vi "STS_spectroscopy_V1.vi"(6 "Internal use":string, 7 "Grid param":T1 {"height (m)" format="%#_6p"; "width (m)" format="%#_6p"; "center Y (m)" format="%#_6p"; "center X (m)" format="%#_6p"}, 8 "Error in (no error)":errorcluster, 9 "Points Y/Index Y":i32, 10 "Points X/Index X":i32, 11 "Method":enum16{"init", "run", "end"}(ring)=enum."end") -> (0 "Error out":errorcluster)   [LabVIEW 2014]
doc: "Example of a measurement VI to be used in the \"Experiments on a Grid\" tool as external VI.\n\nThis example measure the topography and spectroscopy data. The spectroscopy measurements are taken on a subgrid. The data are saved to a sxm and a binary file.\n\n- Nanonis Programming Interface -"
uses:
  <userlib>/Nanonis Prog Interface V5/Scan/Grid/LinePatternGet.vi
  <userlib>/Nanonis Prog Interface V5/Scan/Grid/GridPatternGet.vi
  <userlib>/Nanonis Prog Interface V5/Scan/Grid/CloudPatternGet.vi
  <userlib>/Nanonis Prog Interface V5/Nanonis Prog Interface.lvlib
panel:
  out "Status 2":string="finishing"
  in  "Lockin delay [ms]":u32
  in  "Z Controller ON/OFF":bool
  in  "type":u16(ring)=1 items=["Line", "Grid", "Cloud"]
  in  "Lockin ON/OFF":bool
  in  "Correct Drift":bool=TRUE
  in  "Email when finished":string="cornelius.krull@monash.edu, dhaneesh.gopalakrishnan@monash.edu"
  in  "STS z offset":dbl format="%#_6p"
  out "ETA":timestamp=timestamp(3582621546.85837 s since 1904-01-01)
  out "remaining":dbl=19834.093046092985 format="%<%H:%M:%S>t"
  out "Progress":u8(slide)=5 scale=0.0..100.0 scale format="%#.1g"
  out "total Points":i32=576
  in  "preSTS delay [ms]":u32=3
  in  "STS Bias":dbl=-3.4 format="%#_6p"
  in  "Move Bias":dbl=-3.4 format="%#_6p"
  in  "Move Current":dbl=5e-11 format="%#_6p"
  in  "Imaging Bias":dbl=-3.4 format="%#_6p"
  in  "max applied Drift Correction":i32=20 min=1 max=100 step=1 format="%.0p"
  in  "Correlate":u16(ring) items=["first Frame", "successive Frames"]
  out "Topo Images taken":i32
  in  "Increment":i32=40
  in  "Threshold":i32=2 min=1 step=1
  in  "tip Speed (m/s)":sgl=1e-08 format="%.2p"
  out "X drift":i32
  out "Y drift":i32
  out "Last Drift detected":i32
  in  "MaxImagesBack":i32=2
  in  "Channel index (0-23)":u8(ring) items=["Current"=0, "Z (m)"=14]
  in  "File name":string="DCA_cluster_STS_Grid"
  in  "STS Current":dbl=5e-11 format="%#_6p"
  in  "Imaging Current":dbl=5e-11 format="%#_6p"
  in  "zdrift \nDuration (s)":dbl
  in  "Correct z drift":bool
  out "Status":string="finishing"
  in  "Drift correction Pixels":i32=256 caption="Topo Pixels"
  out "Y Offset":dbl format="%#_6p"
  out "X Offset":dbl format="%#_6p"
  out "Points taken":dbl=30.0
  in  "Drift Correction every":i32=40
  in  "Y subgrid spacing":u16=1
  in  "X subgrid spacing":u16=1
  # "GRID points"
  # "Increase this if no Drift was detected for \na certain number of images"
  # "%"
  # "time (HH:MM:SS)"
  # "images back"
  # "% of image size"
  # "<--Z Cont. Needs to be off"
  # "RUN smart tilt before starting the GRID | Img Angle = 0"
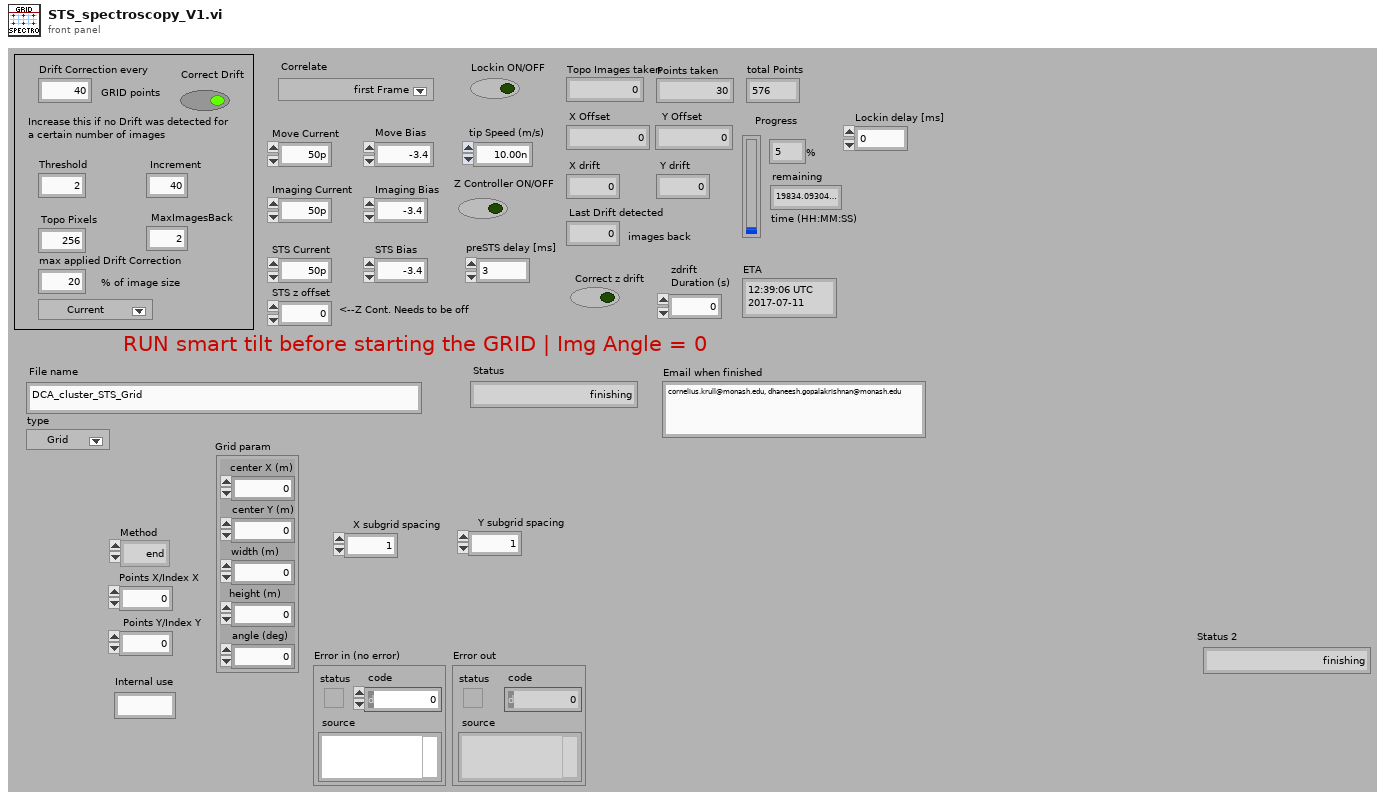
[diagram p1: front panel]
types:
  T1 = cluster{"center X (m)":sgl, "center Y (m)":sgl, "width (m)":sgl, "height (m)":sgl, "angle (deg)":sgl}
  T2 = cluster{"Drift correction Pixels":i32, "Imaging Current":dbl, "STS Current":dbl, "MaxImagesBack":i32, "tip Speed (m/s)":sgl, "Threshold":i32, "Increment":i32, "Correlate":u16, "max applied Drift Correction":i32, "Imaging Bias":dbl, "Move Current":dbl, "Move Bias":dbl, "STS Bias":dbl, "preSTS delay [ms]":u32, "STS z offset":dbl, "Correct Drift":bool, "Lockin ON/OFF":bool}
  T3 = cluster{"center X":sgl, "center Y":sgl, "angle":sgl, "width":sgl, "height":sgl, "# pixels":i32, "# lines":i32}
  T4 = cluster{"Name":string, "Calibration":sgl, "Offset":sgl, "Channel index":i32}[]
  T5 = cluster{"up/down":bool, "time/line":sgl, "start time":timestamp, "end time":timestamp}
  T6 = cluster{"Z averaging time (s)":sgl, "Z offset (m)":sgl, "Initial settling time (s)":sgl}
  T7 = cluster{"Max. slew rate (V/s)":sgl, "Settling time (s)":sgl, "Integration time (s)":sgl}
  T8 = cluster{"End settling time (s)":sgl, "Z control time (s)":sgl}
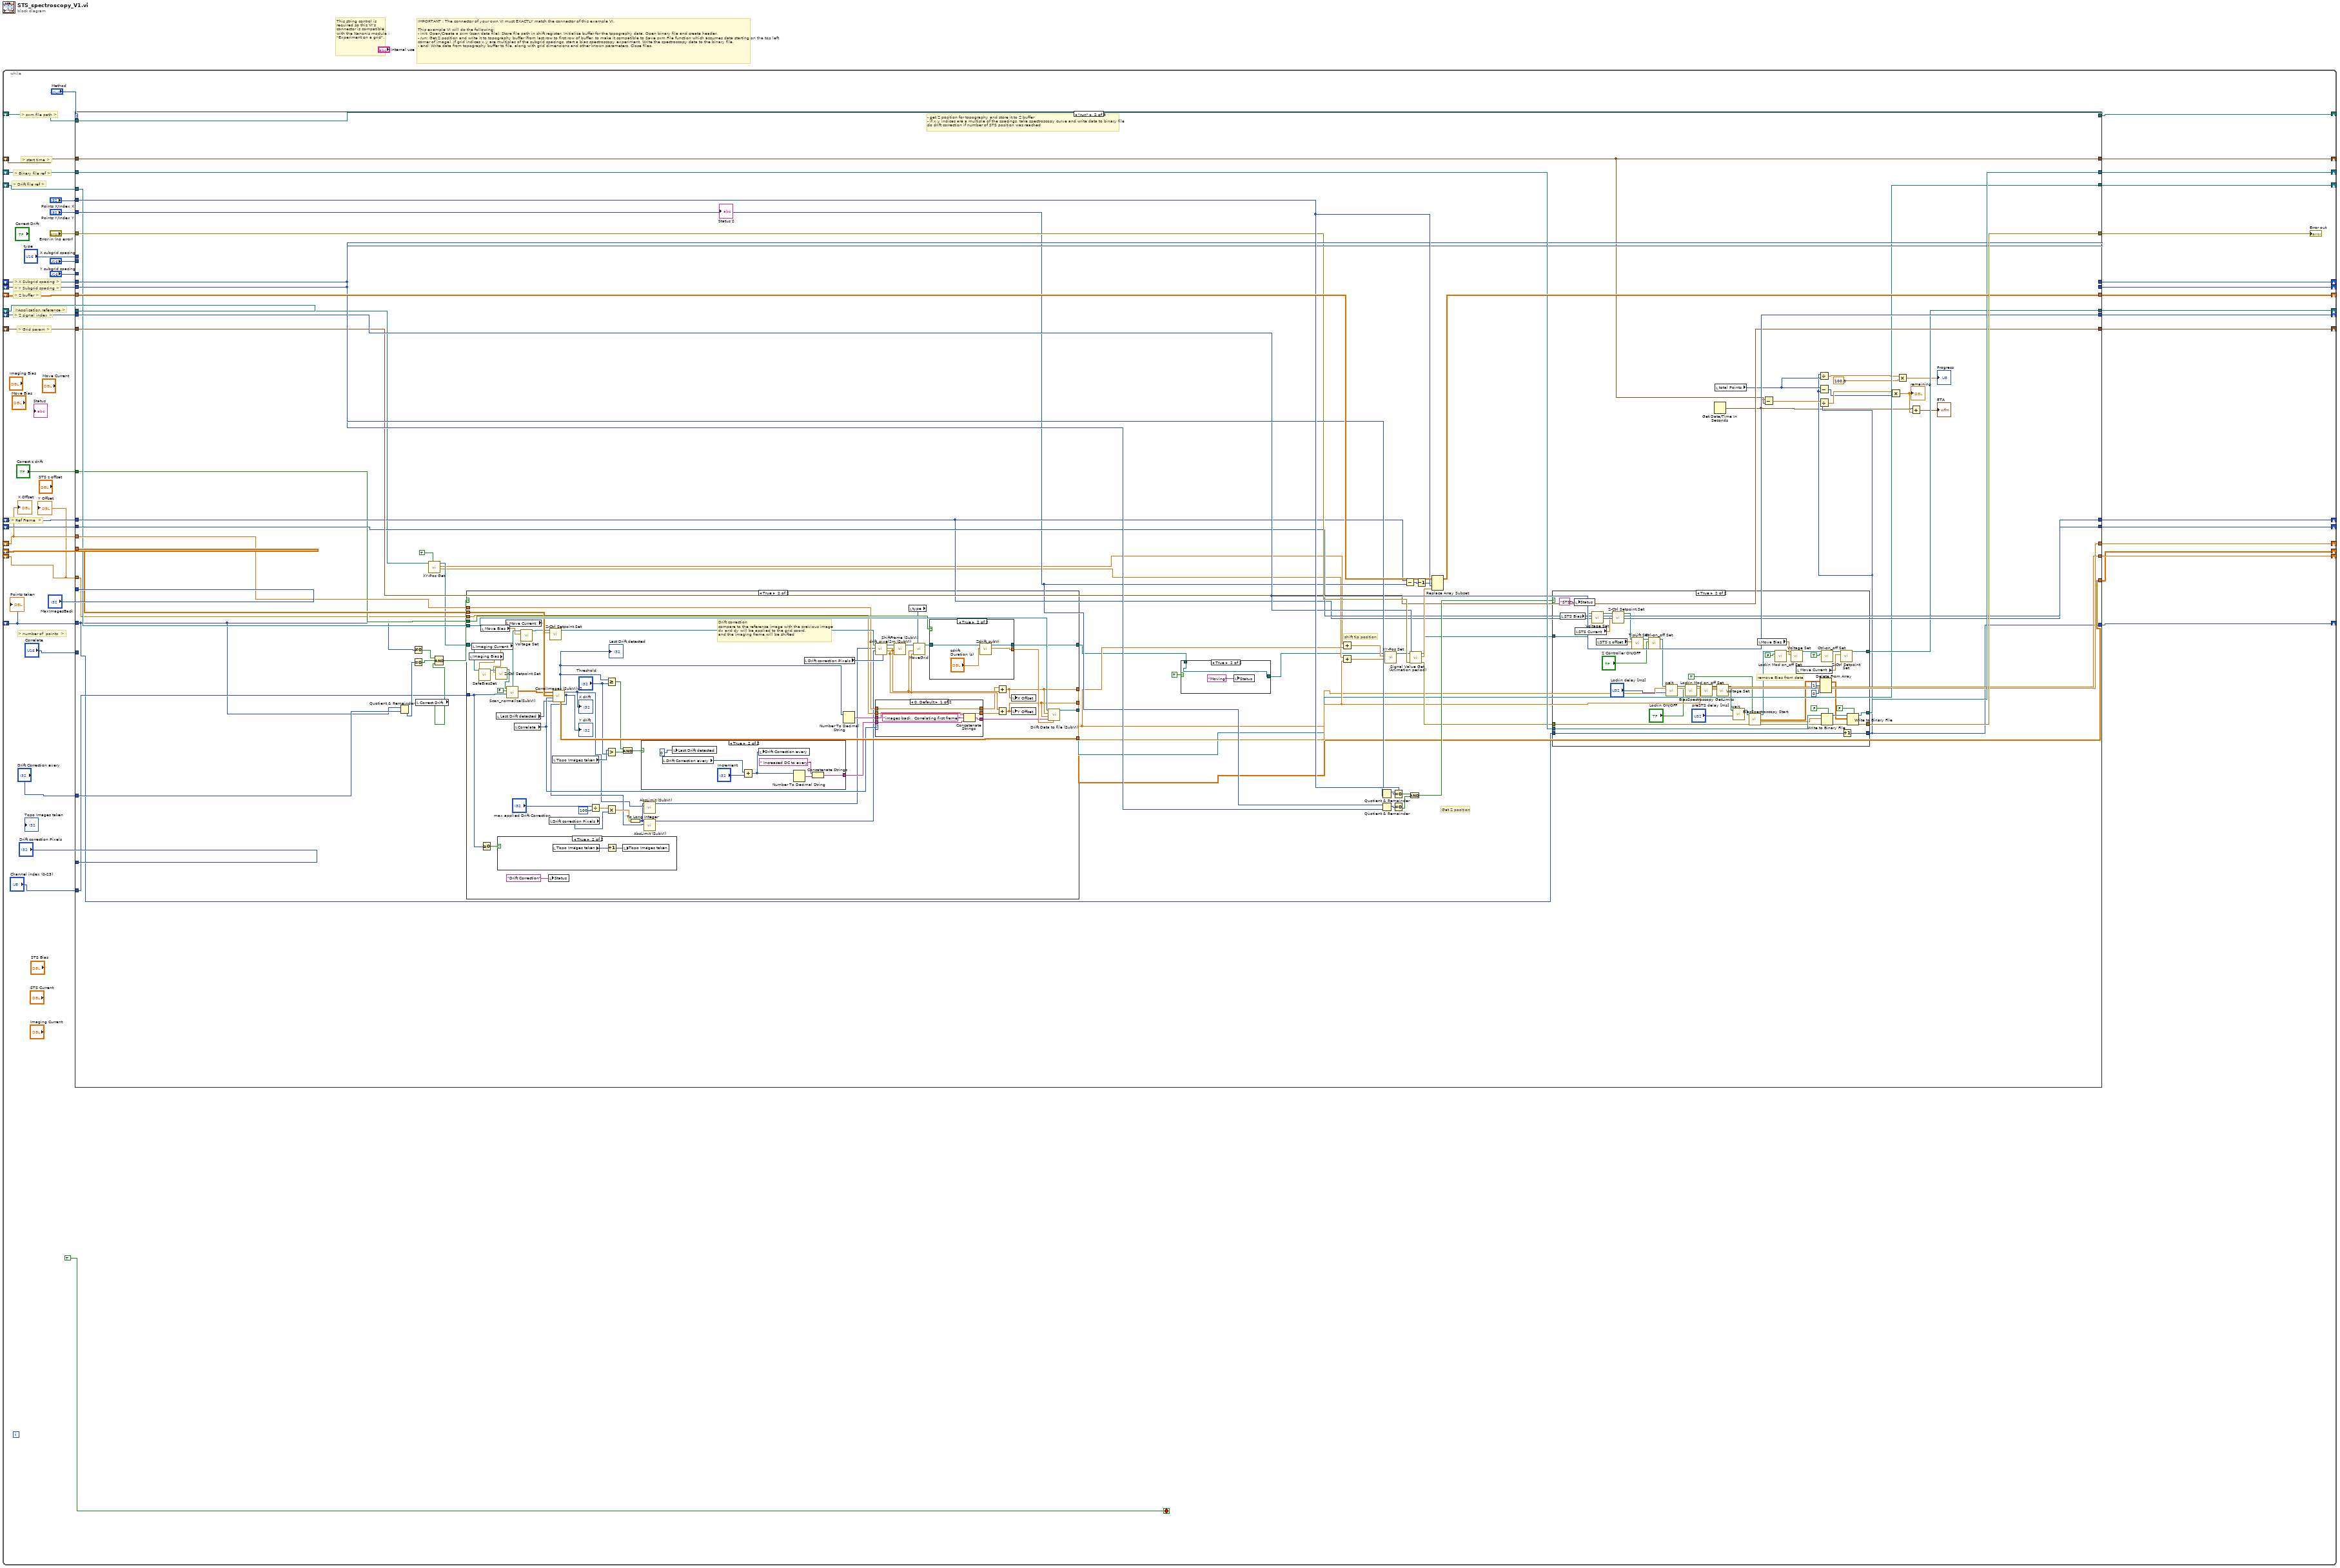
[diagram p0: block diagram]
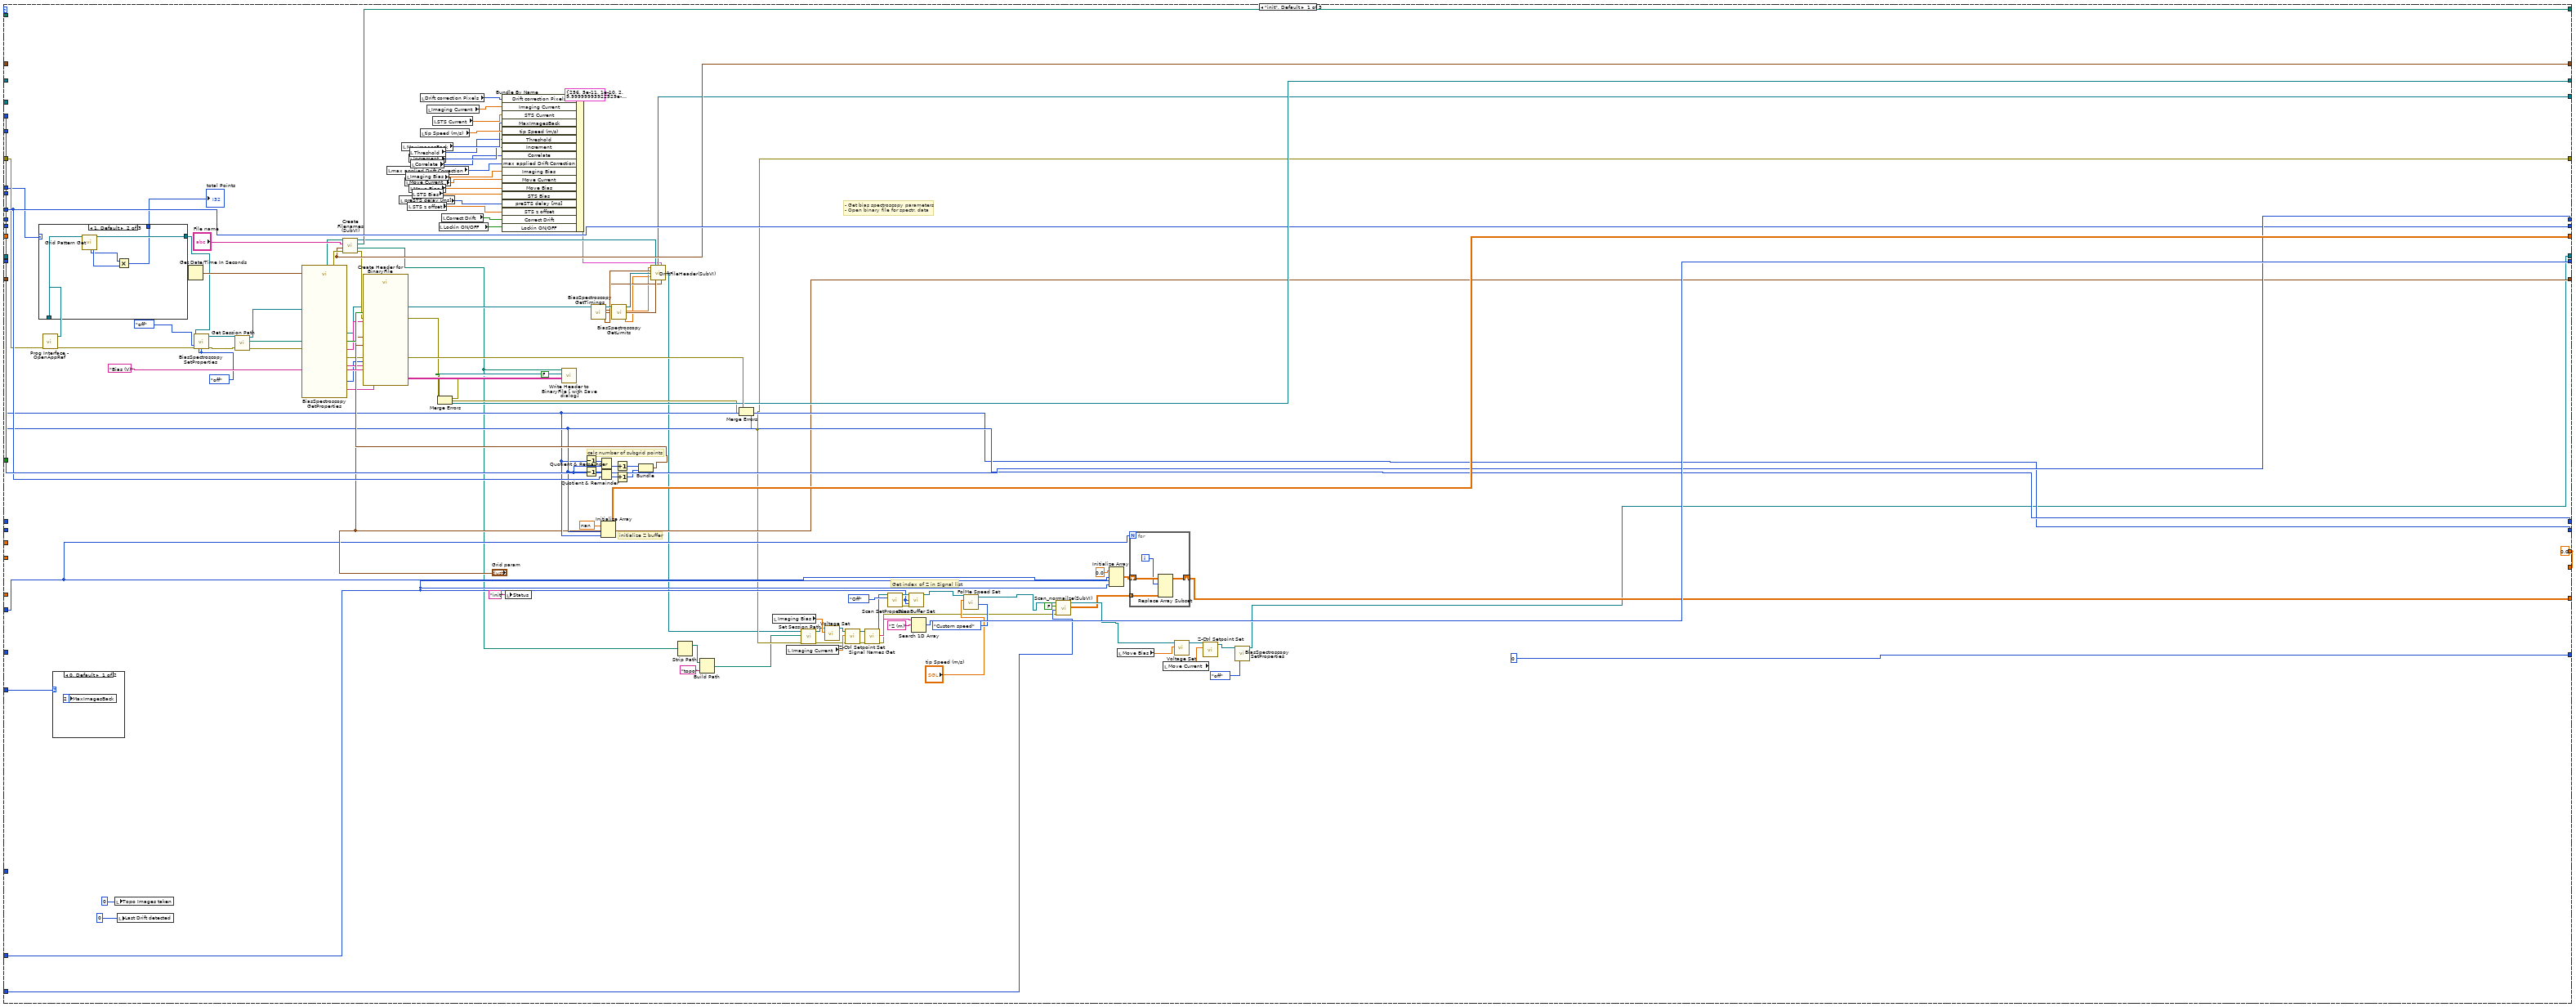
[diagram p2: hidden frame]
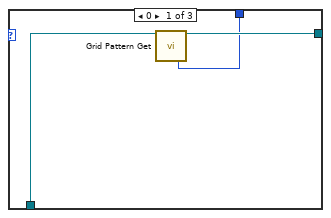
[diagram p3: hidden frame]
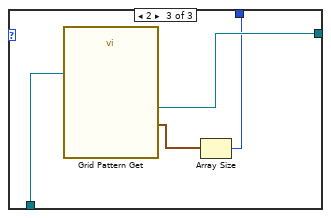
[diagram p4: hidden frame]
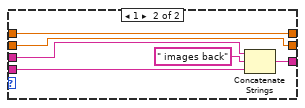
[diagram p8: hidden frame]
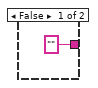
[diagram p10: hidden frame]
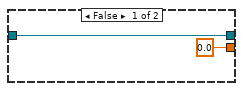
[diagram p11: hidden frame]
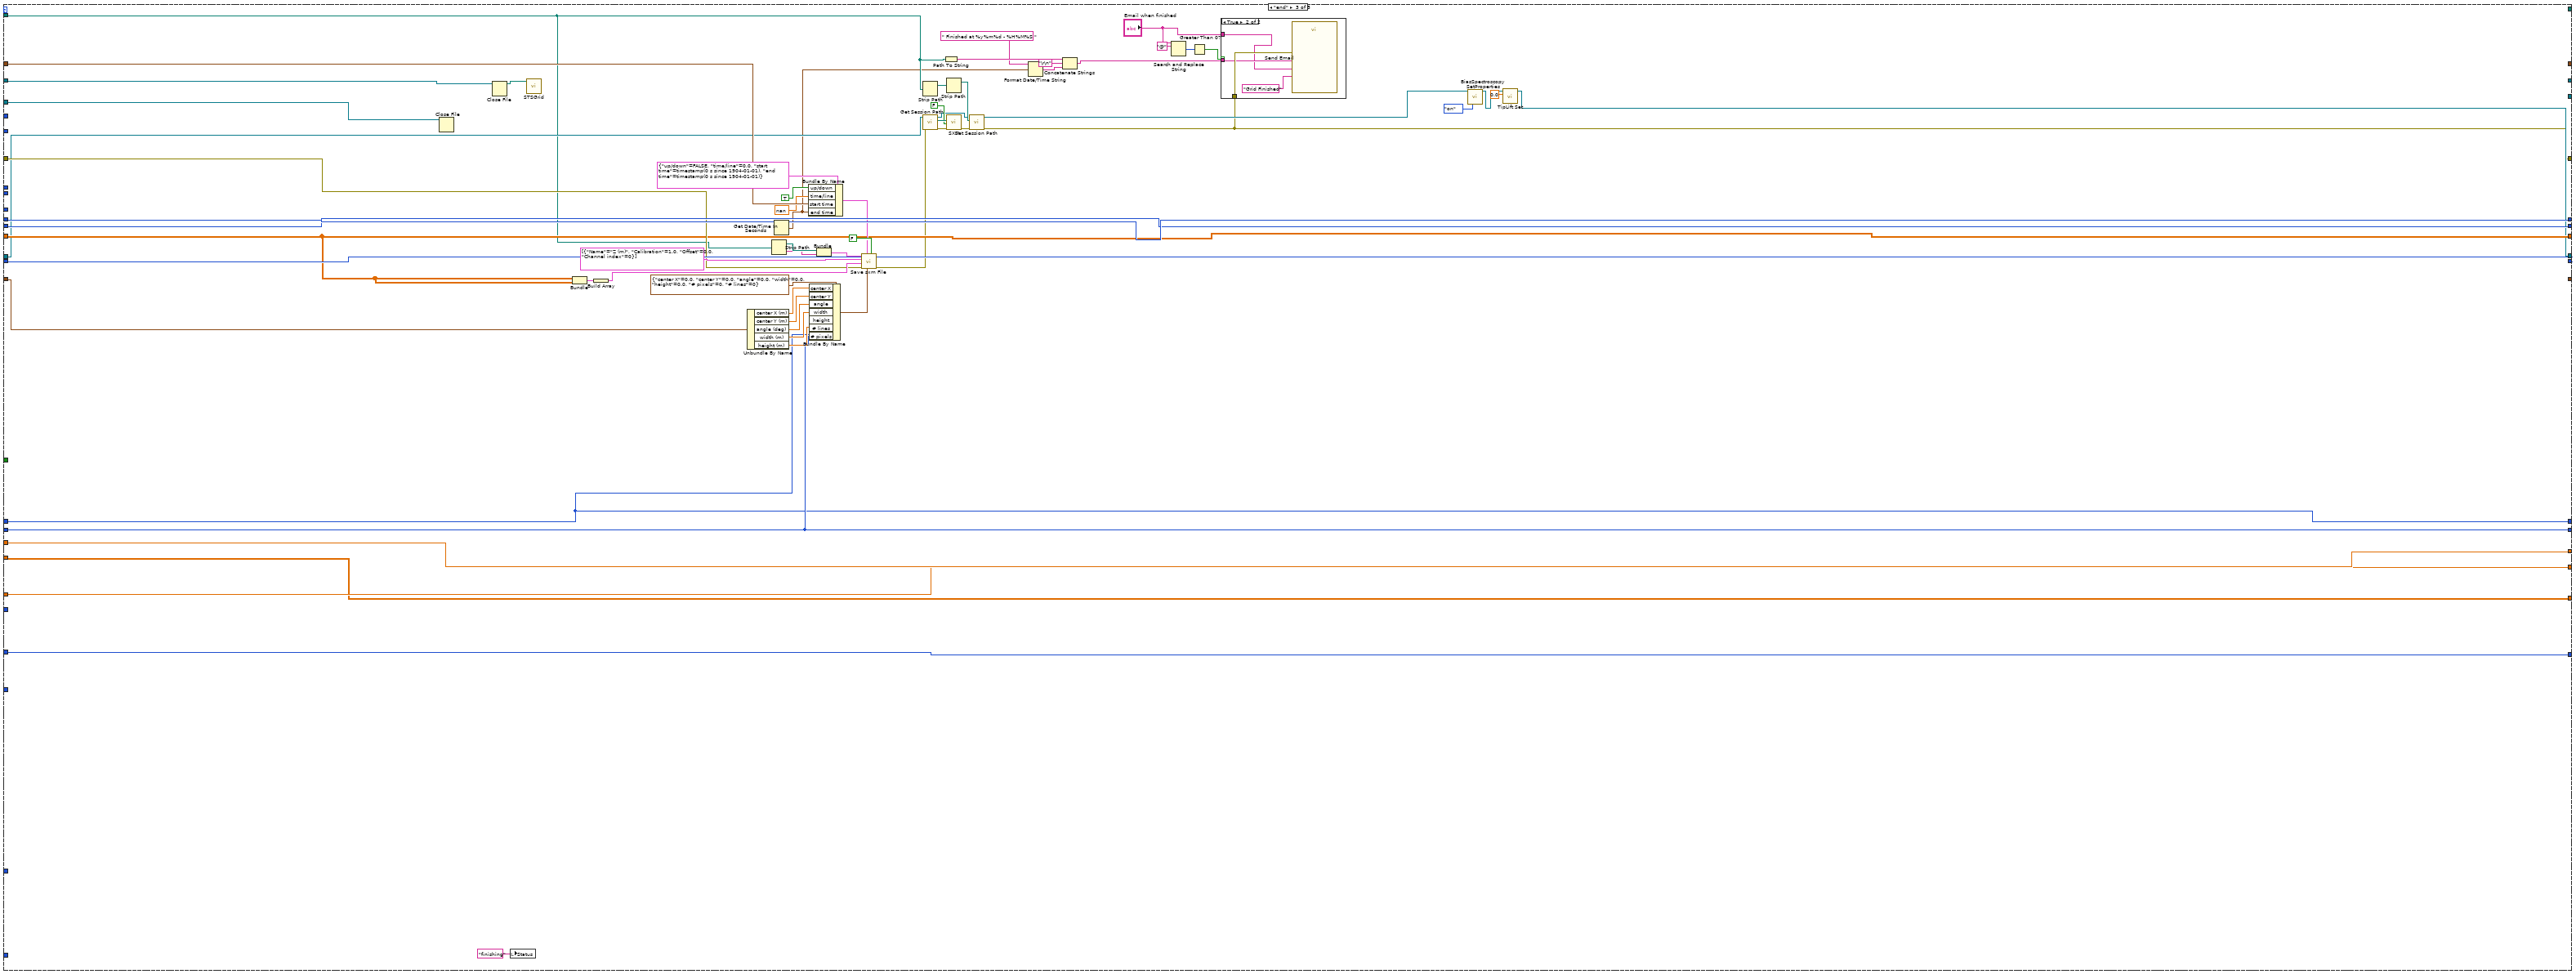
[diagram p13: hidden frame]
diagram:
  # "This string control is required so this VI's connector is compatible with the Nanonis module : \"Experiment on a grid\"."
  # "IMPORTANT : The connector of your own VI must EXACTLY match the connector of this example VI.\n\nThis example VI will do the following:\n- init: Open/Create a sxm (scan data file). Store file path in shift register. Initialize buffer for the topography data. Open binary file and create header.\n- run: Get Z position and write it to topography buffer (from last row to first row of buffer, to make it compatible to Save sxm File function which assumes data starting on the top left corner of image). If grid indices x,y are multiples of the subgrid spacings, start a bias spectroscopy experiment. Write the spectroscopy data to the binary file.\n- end: Write data from topography buffer to file, along with grid dimensions and other known parameters. Close files."
  n1 = while {
    shift-right: [w22] -> _
    shift-left: _ -> [w45]
    shift-right: [w40] -> _
    shift-left: _ -> [w39]
    shift-right: [w37] -> _
    shift-left: _ -> [w38]
    shift-right: [w36] -> _
    shift-left: _ -> [w35]
    shift-right: [w29] -> _
    shift-left: _ -> [w31]
    shift-right: [w30] -> _
    shift-left: _ -> [w32]
    shift-right: [w28] -> _
    shift-left: _ -> [w27]
    shift-right: [w26] -> _
    shift-left: _ -> [w25]
    shift-right: [w24] -> _
    shift-left: _ -> [w23]
    shift-right: [w21] -> _
    shift-left: _ -> [w20]
    shift-right: [w19] -> _
    shift-left: _ -> [w18]
    shift-right: [w17] -> _
    shift-left: _ -> [w10]
    shift-right: [w16] -> _
    shift-left: _ -> [w9]
    shift-right: [w15] -> _
    shift-left: _ -> [w12]
    shift-right: [w14] -> _
    shift-left: _ -> [w11]
    shift-right: [w7] -> _
    shift-left: _ -> [w6]
    stop <- TRUE stop-if-true
    # "> Drift file ref >"
    # "> number of  points  >"
    # "> Ref Frame  >"
    # "> Grid param >"
    # "> start time >"
    # ">Application reference >"
    # "> Y Subgrid spacing >"
    # "> X Subgrid spacing >"
    # "> Z signal index >"
    # "> Binary file ref >"
    # "> Z buffer >"
    # "> sxm file path >"
    n2 = case shown="\"run\"" "Method" {
      tunnel: [w127 w248 _] -> w22
      tunnel: w45 -> [_ w248 w409]
      tunnel: "Error in (no error)" -> [w129 w234 w436]
      tunnel: [w52 w247 w390] -> w43
      tunnel: "Points X/Index X" -> [w141 w242 _]
      tunnel: "Points Y/Index Y" -> [w142 w227 _]
      tunnel: [w165 w245 w425] -> w40
      tunnel: w39 -> [_ w246 w425]
      tunnel: w38 -> [_ w244 w418]
      tunnel: [w157 w243 _] -> w37
      tunnel: [w155 w232 w450] -> w36
      tunnel: w35 -> [_ w232 w450]
      tunnel: "X subgrid spacing" -> [w154 _ _]
      tunnel: "Y subgrid spacing" -> [w153 _ _]
      tunnel: w32 -> [_ w236 w449]
      tunnel: w31 -> [_ w235 w448]
      tunnel: [w154 w236 w449] -> w30
      tunnel: [w153 w235 w448] -> w29
      tunnel: [w91 w220 w396] -> w28
      tunnel: w27 -> [_ w203 w413]
      tunnel: ["Grid param" w230 _] -> w26
      tunnel: w25 -> [_ w230 w435]
      tunnel: [w126 w194 _] -> w24
      tunnel: w23 -> [_ w194 w443]
      tunnel: [w142 w228 w426] -> w21
      tunnel: w20 -> [_ w228 w426]
      tunnel: [w141 w229 w427] -> w19
      tunnel: w18 -> [_ w229 w427]
      tunnel: [w138 w210 w424] -> w17
      tunnel: [w138 w215 w422] -> w16
      tunnel: [w122 w209 w419] -> w15
      tunnel: [0 w192 w423] -> w14
      tunnel: w11 -> [_ w206 w423]
      tunnel: "Drift Correction every" -> [_ w223 _]
      tunnel: w12 -> [_ w214 w419]
      tunnel: w10 -> [_ w221 w424]
      tunnel: w9 -> [_ w207 w422]
      tunnel: "Drift correction Pixels" -> [w121 _ _]
      tunnel: [w86 w212 _] -> w7
      tunnel: w6 -> [_ w213 w420]
      tunnel: "Correct z drift" -> [_ w211 _]
      tunnel: "Channel index (0-23)" -> [w60 w208 _]
      tunnel: "MaxImagesBack" -> [w120 _ _]
      tunnel: "Correlate" -> [w102 _ _]
      tunnel: "type" -> [w54 _ _]
      frame "init", Default {
        w88 = enum16{"no change", "on", "off"}."off" ("Save dialog")
        w138 = 0.0
        # "- Get bias spectroscopy parameters\n- Open binary file for spectr. data"
        # "initialize Z buffer"
        # "calc number of subgrid points"
        # "Get index of Z in Signal list"
        n3 = call <userlib>:"Prog Interface - OpenAppRef.vi"("Error in (no error)"=w129) -> ("Error out"=w108:errorcluster, "Application reference"=w93:refnum<vi>)  [unwired: 5 in]
        n4 = case shown="1, Default" w54 {
          tunnel: w93 -> [w168 w173 w177]
          tunnel: [w167 w172 w176] -> w92
          tunnel: [w166 w169 w174] -> w53
          frame 0 {
            n5 = call-poly <userlib>:"Grid Pattern Get.vi"("Application ref in"=w168) -> ("Points"=w166:i32, "Application ref out"=w167:refnum<vi>)  [unwired: 12 in, 5 out]
          }
          frame 1, Default {
            n6 = call-poly <userlib>:"Grid Pattern Get.vi"("Application ref in"=w173) -> ("Points Y"=w170:i32, "Points X"=w171:i32, "Application ref out"=w172:refnum<vi>)  [unwired: 10 in, 6 out]
            n7 = Multiply(x=w170, y=w171) -> (x*y=w169:i32)
          }
          frame 2 {
            n8 = call-poly <userlib>:"Grid Pattern Get.vi"("Application ref in"=w177) -> ("Application ref out"=w176:refnum<vi>, "Cloud data"=w175:cluster{"X":sgl, "Y":sgl}[])  [unwired: 16 in, 1 out]
            n9 = Array Size(array=w175) -> (size(s)=w174:i32)
          }
        }
        "total Points" <- w53
        n10 = case shown="0, Default" w102 {
          frame 0, Default {
            n11 = local write "MaxImagesBack"(2 ("StepsBack")) -> ()
          }
          frame 1 {
          }
        }
        n12 = local write "Topo Images taken"(0 ("Images taken")) -> ()
        n13 = local write "Last Drift detected"(0 ("Last Drift detected")) -> ()
        n14 = Get Date/Time In Seconds() -> (seconds since 1Jan1904=w126:timestamp)
        n15 = call <userlib>:"BiasSpectroscopy SetProperties.vi"("Application ref in"=w92, "Autosave (no change)"=enum16{"no change", "on", "off"}."off", "Error in (no error)"=w108, "Z-Controller hold (no change)"=w88, "Save dialog"=w88) -> ("Application ref out"=w105:refnum<vi>, "Error out"=w104:errorcluster)  [unwired: 9 in]
        n16 = call <userlib>:"Get Session Path.vi"("error in (no error)"=w104, "Application ref in"=w105) -> ("error out"=w128:errorcluster, "Session path"=w112:path, "Application ref out"=w106:refnum<vi>)  [unwired: 7 in]
        n17 = call <userlib>:"BiasSpectroscopy GetProperties.vi"("Application ref in"=w106) -> ("Backward sweep"=w161:bool, "Application ref out"=w115:refnum<vi>, "Number of points"=w144:i32, "Channels"=w143:string[], "Parameters"=w159:string[], "Fixed parameters"=w146:string[], "Error out"=w158:errorcluster)  [unwired: 6 in, 2 out]
        n18 = call "Create Filenames (SubVI).vi"("error in (no error)"=w128, "seconds since 1Jan1904"=w126, "File name"="File name", "Session path"=w112) -> ("error out"=w116:errorcluster, "binFilePath"=w109:path, "topoFilePath"=w127:path, "Drift File out"=w87:refnum<file>)  [unwired: 4 in]
        n19 = local read "max applied Drift Correction"() -> (w68:i32)
        n20 = local read "preSTS delay [ms]"() -> (w63:u32)
        n21 = local read "MaxImagesBack"() -> (w72:i32)
        n22 = local read "Move Current"() -> (w66:dbl)
        n23 = local read "Imaging Bias"() -> (w67:dbl)
        n24 = local read "STS z offset"() -> (w62:dbl)
        n25 = local read "Increment"() -> (w70:i32)
        n26 = local read "Move Bias"() -> (w65:dbl)
        n27 = local read "Threshold"() -> (w71:i32)
        n28 = local read "Correlate"() -> (w69:u16)
        n29 = local read "STS Bias"() -> (w64:dbl)
        n30 = local read "Drift correction Pixels"() -> (w77:i32)
        n31 = local read "tip Speed (m/s)"() -> (w74:sgl)
        n32 = local read "Imaging Current"() -> (w76:dbl)
        n33 = local read "STS Current"() -> (w75:dbl)
        n34 = local read "Lockin ON/OFF"() -> (w73:bool)
        n35 = local read "Correct Drift"() -> (w61:bool)
        n36 = Bundle By Name(cluster=T2 {"Drift correction Pixels"=256, "Imaging Current"=5e-11, "STS Current"=1e-10, "MaxImagesBack"=2, "tip Speed (m/s)"=1e-08, "Threshold"=2, "Increment"=64, "Correlate"=0, "max applied Drift Correction"=20, "Imaging Bias"=-0.02, "Move Current"=1.5e-11, "Move Bias"=-0.02, "STS Bias"=0.1, "preSTS delay [ms]"=1000, "STS z offset"=-1.7e-10, "Correct Drift"=TRUE, "Lockin ON/OFF"=TRUE} ("Drift Correction"), "Drift correction Pixels"=w77, "Imaging Current"=w76, "STS Current"=w75, "MaxImagesBack"=w72, "tip Speed (m/s)"=w74, "Threshold"=w71, "Increment"=w70, "Correlate"=w69, "max applied Drift Correction"=w68, "Imaging Bias"=w67, "Move Current"=w66, "Move Bias"=w65, "STS Bias"=w64, "preSTS delay [ms]"=w63, "STS z offset"=w62, "Correct Drift"=w61, "Lockin ON/OFF"=w73) -> (w79:T2)
        n37 = local write "Status"("init" ("Status")) -> ()
        n38 = Decrement(x=w141) -> (x-1=w152:i32)
        n39 = Decrement(x=w142) -> (x-1=w151:i32)
        n40 = call <userlib>:"BiasSpectroscopy GetTimings.vi"("Application ref in"=w115) -> ("Application ref out"=w119:refnum<vi>, "Initialization"=w82:T6, "Sweep Timing"=w83:T7, "End of Sweep"=w84:T8)  [unwired: 10 in, 1 out]
        n41 = Quotient & Remainder(x=w152, y=w154) -> (floor(x/y)=w150:i32)  [unwired: 1 out]
        n42 = Quotient & Remainder(x=w151, y=w153) -> (floor(x/y)=w149:i32)  [unwired: 1 out]
        n43 = Initialize Array(sgl nan ("element"), w142, w141) -> (w165:sgl[][])
        n44 = call <userlib>:"BiasSpectroscopy GetLimits.vi"("Application ref in"=w119) -> ("End value (V)"=w80:sgl, "Start value (V)"=w81:sgl, "Application ref out"=w85:refnum<vi>)  [unwired: 5 in, 1 out]
        n45 = Increment(x=w150) -> (x+1=w148:i32)
        n46 = Increment(x=w149) -> (x+1=w147:i32)
        n47 = Bundle(w148, w147) -> (w160:cluster{i32, i32})  [unwired: 1 in]
        n48 = call <userlib>:"Create Header for BinaryFile.vi"("Grid points"=w160, "Grid param"="Grid param", "Fixed parameters"=w146, "Backward sweep"=w161, "Sweep signal"="Bias (V)" ("Sweep Signal"), "Parameters"=w159, "Channels"=w143, "Points per sweep"=w144) -> ("Header (fixed attributes)"=w163:string[][])  [unwired: 3 in]
        n49 = call <userlib>:"Write Header to BinaryFile [ with Save dialog].vi"("Fixed Attributes"=w163, "Show Dialog? (T)"=FALSE, "Filename"=w109) -> ("Error out"=w117:errorcluster, "File ref"=w157:refnum<file>)  [unwired: 5 in, 2 out]
        n50 = Merge Errors(w117, w116) -> (w118:errorcluster)
        n51 = call "DriftFileHeader(SubVI).vi"("Start value (V)"=w81, "Byte Stream File in"=w87, "Drift Correction"=w79, "End of Sweep"=w84, "Application ref in"=w85, "End value (V)"=w80, "Sweep Timing"=w83, "Initialization"=w82) -> ("Byte Stream File out"=w86:refnum<file>, "Application ref out"=w49:refnum<vi>)  [unwired: 6 in]
        n52 = Strip Path(path=w109) -> (stripped path=w111:path)  [unwired: 1 out]
        n53 = Build Path(base path=w111, name or relative path="topo") -> (appended path=w51:path)
        n54 = Merge Errors(w158, w118) -> (w52:errorcluster)
        n55 = local read "Imaging Bias"() -> (w95:dbl)
        n56 = local read "Imaging Current"() -> (w94:dbl)
        n57 = call <userlib>:"Set Session Path.vi"("error in (no error)"=w52, "Session Folder"=w51, "Application ref in"=w49) -> ("error out"=w50:errorcluster, "Application ref out"=w48:refnum<vi>)  [unwired: 7 in]
        n58 = call <userlib>:"Voltage Set.vi"("Bias (V)"=w95, "Application ref in"=w48) -> ("Application ref out"=w98:refnum<vi>)  [unwired: 8 in, 1 out]
        n59 = call <userlib>:"Z-Ctrl Setpoint Set.vi"("error in (no error)"=w50, "Z Controller setpoint"=w94, "Application ref in"=w98) -> ("error out"=w130:errorcluster, "Application ref out"=w131:refnum<vi>)  [unwired: 7 in]
        n60 = call <userlib>:"Signal Names Get.vi"("error in (no error)"=w130, "Application ref in"=w131) -> ("error out"=w57:errorcluster, "Signals Names"=w145:string[], "Application ref out"=w134:refnum<vi>)  [unwired: 5 in]
        n61 = call <userlib>:"Scan SetProperties.vi"("Application ref in"=w134, "Continuous scan"=enum16{"No change", "On", "Off"}."Off") -> ("Application ref out"=w136:refnum<vi>, "Error out"=w135:errorcluster)  [unwired: 12 in]
        n62 = call <userlib>:"ScanBuffer Set.vi"("Application ref in"=w136, "Pixels"=w121, "Lines"=w121, "error in (no error)"=w135) -> ("Application ref out"=w100:refnum<vi>)  [unwired: 10 in, 1 out]
        n63 = Search 1D Array(1D array=w145, element="Z (m)") -> (index of element=w155:i32)  [unwired: 1 in]
        n64 = call <userlib>:"FolMe Speed Set.vi"("Speed Setting (Custom)"=enum32{"Scan speed", "Custom speed"}."Custom speed", "Speed (m/s)"="tip Speed (m/s)", "Application ref in"=w100) -> ("Application ref out"=w59:refnum<vi>)  [unwired: 5 in, 1 out]
        n65 = call "Scan_normailze(SubVI).vi"("error in (no error)"=w57, "Channel index (0-23)"=w60, "Normalization"=FALSE ("Boolean"), "Application in"=w59) -> ("Array"=w56:dbl[][], "Application out"=w58:refnum<vi>)  [unwired: 5 in, 1 out]
        n66 = Initialize Array(0.0 ("element"), w120, w121, w121) -> (w123:dbl[][][])
        n67 = local read "Move Bias"() -> (w97:dbl)
        n68 = for {
          N: w120 -> [_]
          tunnel: w56 -> [w181]
          shift-right: [w180] -> w122
          shift-left: w123 -> [w182]
          i -> [w179]
          n69 = Replace Array Subset(array=w182, new element=w181, index (dim 0)=w179) -> (w180:dbl[][][])  [unwired: 2 in]
        }
        n70 = local read "Move Current"() -> (w96:dbl)
        n71 = call <userlib>:"Voltage Set.vi"("Bias (V)"=w97, "Application ref in"=w58) -> ("Application ref out"=w99:refnum<vi>)  [unwired: 8 in, 1 out]
        n72 = call <userlib>:"Z-Ctrl Setpoint Set.vi"("Z Controller setpoint"=w96, "Application ref in"=w99) -> ("Application ref out"=w90:refnum<vi>)  [unwired: 8 in, 1 out]
        n73 = call <userlib>:"BiasSpectroscopy SetProperties.vi"("Application ref in"=w90, "Z-Controller hold (no change)"=enum16{"no change", "on", "off"}."off") -> ("Application ref out"=w91:refnum<vi>)  [unwired: 12 in, 1 out]
      }
      frame "run" {
        # "shift tip position"
        # "Get Z position"
        # "- get Z position for topography and store it to Z buffer\n- if x,y indices are a multiple of the spacings, take spectroscopy curve and write data to binary file\ndo drift correction if number of STS position was reached"
        n74 = Quotient & Remainder(x=w206, y=w223) -> (x-y*floor(x/y)=w224:i32)  [unwired: 1 out]
        n75 = Not Equal To 0?(x=w206) -> (x != 0?=w204:bool)
        n76 = Equal To 0?(x=w224) -> (x = 0?=w222:bool)
        n77 = local read "Correct Drift"() -> (w186:bool)
        n78 = call <userlib>:"XY-Pos Get.vi"("Wait for newest data (F=False)"=TRUE, "Application ref in"=w203) -> ("Y (m)"=w199:sgl, "X (m)"=w200:sgl, "Application ref out"=w202:refnum<vi>)  [unwired: 5 in, 1 out]
        n79 = Compound Arithmetic op=AND(w204, w222, w186) -> (w205:bool)
        n80 = case shown="True" w205 {
          tunnel: w202 -> [w256 w266]
          tunnel: [w256 w308] -> w185
          tunnel: w214 -> [w253 w303]
          tunnel: [w255 w306] -> w210
          tunnel: [w254 w305] -> w215
          tunnel: w221 -> [w255 w282]
          tunnel: w207 -> [w254 w280]
          tunnel: [w253 w299] -> w209
          tunnel: w213 -> [w252 w311]
          tunnel: [w252 w310] -> w212
          tunnel: w211 -> [_ w307]
          tunnel: w208 -> [_ w286]
          frame False {
          }
          frame True {
            # "Drift correction \ncompare to the reference image with the previous image \ndx and dy will be applied to the grid coord, \nand the imaging frame will be shifted"
            n81 = local read "Imaging Bias"() -> (w264:dbl)
            n82 = local read "Imaging Current"() -> (w263:dbl)
            n83 = call "SafeBiasSet.vi"("Application ref in"=w266, "Bias (V)"=w264) -> ("Application ref out"=w265:refnum<vi>)  [unwired: 7 in, 1 out]
            n84 = local read "Move Bias"() -> (w260:dbl)
            n85 = Greater Or Equal To 0?(x=w286) -> (x >= 0?=w285:bool)
            n86 = call <userlib>:"Z-Ctrl Setpoint Set.vi"("Z Controller setpoint"=w263, "Application ref in"=w265) -> ("Application ref out"=w304:refnum<vi>)  [unwired: 8 in, 1 out]
            n87 = local read "Last Drift detected"() -> (w277:i32)
            n88 = case shown="True" w285 {
              frame False {
              }
              frame True {
                n89 = local read "Topo Images taken"() -> (w326:i32)
                n90 = Increment(x=w326) -> (x+1=w325:i32)
                n91 = local write "Topo Images taken"(w325) -> ()
              }
            }
            n92 = local read "Move Current"() -> (w259:dbl)
            n93 = call "Scan_normailze(SubVI).vi"("Channel index (0-23)"=w286, "Normalization"=FALSE ("Boolean"), "Application in"=w304) -> ("Array"=w300:dbl[][], "Application out"=w261:refnum<vi>)  [unwired: 6 in, 1 out]
            n94 = local read "Correlate"() -> (w283:u16)
            n95 = call <userlib>:"Voltage Set.vi"("Bias (V)"=w260, "Application ref in"=w261) -> ("Application ref out"=w262:refnum<vi>)  [unwired: 8 in, 1 out]
            n96 = local write "Status"("Drift Correction" ("Status")) -> ()
            n97 = local read "Drift correction Pixels"() -> (w274:i32)
            n98 = call <userlib>:"Z-Ctrl Setpoint Set.vi"("Z Controller setpoint"=w259, "Application ref in"=w262) -> ("Application ref out"=w295:refnum<vi>)  [unwired: 8 in, 1 out]
            n99 = local read "Topo Images taken"() -> (w288:i32)
            n100 = call "CorrelImages (SubVI)v2.vi"("last drift detected"=w277, "Correlate"=w283, "Ref Array"=w303, "New Image"=w300) -> ("Y drift"=w271:i32, "X drift"=w268:i32, "Ref Array out"=w299:dbl[][][], "Queue Steps"=w284:i32)  [unwired: 4 in]
            "X drift" <- w268
            "Y drift" <- w271
            "Last Drift detected" <- w284
            n101 = Divide(x="max applied Drift Correction", y=100) -> (x/y=w273:dbl)
            n102 = Greater Or Equal?(x=w284, y="Threshold") -> (x >= y?=w290:bool)
            n103 = Greater?(x=w288, y="Threshold") -> (0:w287:bool)
            n104 = Multiply(x=w273, y=w274) -> (x*y=w275:dbl)
            n105 = And(x=w290, y=w287) -> (x .and. y?=w289:bool)
            n106 = To Long Integer(number=w275) -> (32bit integer=w267:i32)
            n107 = case shown="True" w289 {
              tunnel: ["" w330] -> w291
              frame False {
              }
              frame True {
                n108 = local read "Drift Correction every"() -> (w329:i32)
                n109 = local write "Last Drift detected"(0 ("Last Drift detected")) -> ()
                n110 = Add(x=w329, y="Increment") -> (x+y=w333:i32)
                n111 = local write "Drift Correction every"(w333) -> ()
                n112 = Number To Decimal String(number=w333) -> (decimal integer string=w332:string)  [unwired: 1 in]
                n113 = Concatenate Strings(" Increased DC to every " ("string"), w332) -> (w330:string)
              }
            }
            n114 = call "AbsLimit (SubVI).vi"("in"=w268, "Abslimt"=w267) -> ("Numeric out"=w270:i32)  [unwired: 9 in]
            n115 = call "AbsLimit (SubVI).vi"("in"=w271, "Abslimt"=w267) -> ("Numeric out"=w269:i32)  [unwired: 9 in]
            n116 = local read "Drift correction Pixels"() -> (w296:i32)
            n117 = Number To Decimal String(number=w284) -> (decimal integer string=w302:string)  [unwired: 1 in]
            n118 = call "drift_pixel2m (SubVI).vi"("Application in"=w295, "X drift"=w270, "Y drift"=w269, "Drift correction Pixels"=w296) -> ("Application out"=w294:refnum<vi>, "x drift"=w292:sgl, "y drift"=w293:sgl)  [unwired: 2 in, 1 out]
            n119 = case shown="0, Default" w283 {
              tunnel: w302 -> [w313 w324]
              tunnel: [w318 w323] -> w301
              tunnel: w291 -> [w316 w321]
              tunnel: w282 -> [w314 w320]
              tunnel: [w314 w320] -> w281
              tunnel: w280 -> [w315 w319]
              tunnel: [w315 w319] -> w279
              frame 0, Default {
                n120 = Concatenate Strings(w313, "images back , Correlating first frame " ("string"), w316) -> (w318:string)
              }
              frame 1 {
                n121 = Concatenate Strings(w324, " images back" ("string"), w321) -> (w323:string)
              }
            }
            n122 = call "ShiftFrame (SubVI).vi"("Y shift"=w293, "X shift"=w292, "Application in"=w294) -> ("Application out"=w298:refnum<vi>)  [unwired: 8 in]
            n123 = local read "type"() -> (w257:u16)
            n124 = call "MoveGrid.vi"("type"=w257, "y"=w293, "x"=w292, "Application ref in"=w298) -> ("Application ref out"=w297:refnum<vi>)  [unwired: 6 in, 1 out]
            n125 = case shown="True" w307 {
              tunnel: [0.0 ("z drift") w340] -> w309
              tunnel: w297 -> [w335 w339]
              tunnel: [w335 w338] -> w308
              frame False {
              }
              frame True {
                n126 = call "Zdrift_subVi.vi"("Duration"="zdrift \nDuration (s)", "Application in"=w339) -> ("z drift"=w340:dbl, "Application out"=w338:refnum<vi>)  [unwired: 7 in, 1 out]
              }
            }
            n127 = Add(x=w281, y=w292) -> (x+y=w306:dbl)
            n128 = Add(x=w293, y=w279) -> (x+y=w305:dbl)
            n129 = local write "X Offset"(w306) -> ()
            n130 = local write "Y Offset"(w305) -> ()
            n131 = call "Drift Data to file (SubVI).vi"("z drift"=w309, "Comment"=w301, "y Drift"=w305, "X drift"=w306, "Byte Stream File in"=w311) -> ("Byte Stream File out"=w310:refnum<file>)  [unwired: 6 in]
          }
        }
        n132 = case shown="True" TRUE {
          tunnel: [w249 w250] -> w184
          tunnel: w185 -> [w249 w250]
          frame False {
          }
          frame True {
            n133 = local write "Status"("Moving" ("Status")) -> ()
          }
        }
        n134 = Add(x=w200, y=w210) -> (x+y=w217:dbl)
        n135 = Add(x=w199, y=w215) -> (x+y=w216:dbl)
        n136 = Quotient & Remainder(x=w242, y=w236) -> (x-y*floor(x/y)=w241:i32)  [unwired: 1 out]
        n137 = Quotient & Remainder(x=w227, y=w235) -> (x-y*floor(x/y)=w240:i32)  [unwired: 1 out]
        n138 = call <userlib>:"XY-Pos Set.vi"("Y (m)"=w216, "X (m)"=w217, "Application ref in"=w184) -> ("Application ref out"=w218:refnum<vi>)  [unwired: 5 in, 1 out]
        n139 = Equal To 0?(x=w241) -> (x = 0?=w239:bool)
        n140 = Equal To 0?(x=w240) -> (x = 0?=w238:bool)
        n141 = Subtract(x=w228, y=w227) -> (x-y=w226:i32)
        n142 = And(x=w239, y=w238) -> (x .and. y?=w237:bool)
        n143 = call <userlib>:"Signal Value Get (Animation period).vi"("error in (no error)"=w234, "Signal index (0-47)"=w232, "Application ref in"=w218) -> ("error out"=w233:errorcluster, "Signal value"=w231:sgl, "Application ref out"=w219:refnum<vi>)  [unwired: 5 in]
        n144 = Decrement(x=w226) -> (x-1=w225:i32)
        n145 = Replace Array Subset(array=w246, new element=w231, index (row)=w225, index (col)=w242) -> (w245:sgl[][])
        n146 = case shown="True" w237 {
          tunnel: [w343 w375] -> w247
          tunnel: w244 -> [w344 w389]
          tunnel: [w344 w387] -> w243
          tunnel: w233 -> [w343 w386]
          tunnel: w219 -> [w342 w371]
          tunnel: [w342 w366] -> w220
          tunnel: [w341 w373] -> w192
          tunnel: w206 -> [w341 w374]
          frame False {
            # "Point indices aren't multiple of subgrid spacing\n=> no spectroscopy at this point"
          }
          frame True {
            # "remove Bias from data"
            n147 = local read "STS Bias"() -> (w368:dbl)
            n148 = local write "Status"("STS" ("Status")) -> ()
            n149 = local read "STS Current"() -> (w367:dbl)
            n150 = call <userlib>:"Voltage Set.vi"("Bias (V)"=w368, "Application ref in"=w371) -> ("Application ref out"=w370:refnum<vi>)  [unwired: 8 in, 1 out]
            n151 = local read "STS z offset"() -> (w352:dbl)
            n152 = call <userlib>:"Z-Ctrl Setpoint Set.vi"("Z Controller setpoint"=w367, "Application ref in"=w370) -> ("Application ref out"=w363:refnum<vi>)  [unwired: 8 in, 1 out]
            n153 = call <userlib>:"TipLift Set.vi"("TipLift (m)"=w352, "Application ref in"=w363) -> ("Application ref out"=w350:refnum<vi>)  [unwired: 8 in, 1 out]
            n154 = call <userlib>:"Ctrl-on_off Set.vi"("Z Controller ON/OFF"="Z Controller ON/OFF", "Application ref in"=w350) -> ("Application ref out"=w347:refnum<vi>)  [unwired: 8 in, 1 out]
            n155 = call "wait.vi"("milliseconds to wait"="Lockin delay [ms]", "application reference in"=w347) -> ("application reference out"=w346:refnum<vi>)  [unwired: 8 in, 1 out]
            n156 = call <userlib>:"Lockin Mod on_off Set.vi"("Lockin ON/OFF"="Lockin ON/OFF", "Application ref in"=w346) -> ("Application ref out"=w349:refnum<vi>)  [unwired: 8 in, 1 out]
            n157 = call <userlib>:"BiasSpectroscopy GetLimits.vi"("Application ref in"=w349) -> ("Start value (V)"=w353:sgl, "Application ref out"=w354:refnum<vi>)  [unwired: 5 in, 2 out]
            n158 = call <userlib>:"Voltage Set.vi"("Bias (V)"=w353, "Application ref in"=w354) -> ("Application ref out"=w362:refnum<vi>)  [unwired: 8 in, 1 out]
            n159 = call "wait.vi"("milliseconds to wait"="preSTS delay [ms]", "application reference in"=w362) -> ("application reference out"=w369:refnum<vi>)  [unwired: 8 in, 1 out]
            n160 = call <userlib>:"BiasSpectroscopy Start.vi"("Application ref in"=w369, "Get data (F)"=TRUE ("Get Data (F)"), "Error in (no error)"=w386) -> ("Application ref out"=w358:refnum<vi>, "Data"=w385:sgl[][], "Parameters"=w384:sgl[], "Error out"=w377:errorcluster)  [unwired: 8 in, 1 out]
            n161 = local read "Move Bias"() -> (w365:dbl)
            n162 = call <userlib>:"Lockin Mod on_off Set.vi"("Lockin ON/OFF"=FALSE, "Application ref in"=w358) -> ("Application ref out"=w357:refnum<vi>)  [unwired: 8 in, 1 out]
            n163 = call <userlib>:"Voltage Set.vi"("Bias (V)"=w365, "Application ref in"=w357) -> ("Application ref out"=w360:refnum<vi>)  [unwired: 8 in, 1 out]
            n164 = local read "Move Current"() -> (w364:dbl)
            n165 = Delete From Array(array=w385, length=1, index (row)=0 ("index")) -> (array with subset deleted=w383:sgl[][])  [unwired: 1 in, 1 out]
            n166 = call <userlib>:"Ctrl-on_off Set.vi"("Z Controller ON/OFF"=TRUE, "Application ref in"=w360) -> ("Application ref out"=w359:refnum<vi>)  [unwired: 8 in, 1 out]
            n167 = Write to Binary File(file (use dialog)=w389, data=w384, error in=w377, 5:FALSE ("prepend array or string size? (T)")) -> (refnum out=w388:refnum<file>, error out=w376:errorcluster)  [unwired: 2 in, 1 out]
            n168 = call <userlib>:"Z-Ctrl Setpoint Set.vi"("Z Controller setpoint"=w364, "Application ref in"=w359) -> ("Application ref out"=w366:refnum<vi>)  [unwired: 8 in, 1 out]
            n169 = Increment(x=w374) -> (x+1=w373:i32)
            n170 = Write to Binary File(file (use dialog)=w388, data=w383, error in=w376, 5:FALSE ("prepend array or string size? (T)")) -> (refnum out=w387:refnum<file>, error out=w375:errorcluster)  [unwired: 2 in, 1 out]
          }
        }
        n171 = Get Date/Time In Seconds() -> (seconds since 1Jan1904=w189:timestamp)
        n172 = local read "total Points"() -> (w195:i32)
        n173 = Subtract(x=w189, y=w194) -> (x-y=w193:dbl)
        n174 = Divide(x=w192, y=w195) -> (x/y=w198:dbl)
        n175 = Subtract(x=w195, y=w192) -> (x-y=w190:i32)
        n176 = Divide(x=w193, y=w192) -> (x/y=w191:dbl)
        n177 = Multiply(x=w191, y=w190) -> (x*y=w188:dbl)
        "remaining" <- w188
        n178 = Multiply(x=w198, y=100.0) -> (x*y=→"Progress":dbl)
        n179 = Add(x=w189, y=w188) -> (x+y=→"ETA":timestamp)
      }
      frame "end" {
        n180 = Close File(refnum=w420) -> ()  [unwired: 1 in, 2 out]
        n181 = Close File(refnum=w418) -> (path=w417:path)  [unwired: 1 in, 1 out]
        n182 = local write "Status"("finishing" ("Status")) -> ()
        n183 = call "STSGrid.vi"("Binary Spectroscopy File"=w417) -> ()  [unwired: 11 in]
        n184 = Bundle(w425, w425) -> (w447:cluster{sgl[][], sgl[][]})  [unwired: 1 in]
        n185 = Build Array(w447) -> (w446:cluster{sgl[][], sgl[][]}[])
        n186 = Unbundle By Name(w435) -> ("center X (m)"=w433:sgl, "center Y (m)"=w432:sgl, "angle (deg)"=w431:sgl, "width (m)"=w430:sgl, "height (m)"=w429:sgl)
        n187 = Strip Path(path=w409) -> (stripped path=w439:path, name=w438:string)
        n188 = Get Date/Time In Seconds() -> (seconds since 1Jan1904=w405:timestamp)
        n189 = Bundle By Name(cluster=T5 {"up/down"=FALSE, "time/line"=0.0, "start time"=timestamp(0 s since 1904-01-01), "end time"=timestamp(0 s since 1904-01-01)} ("Scan param"), "up/down"=TRUE, "time/line"=sgl nan ("input 7"), "start time"=w443, "end time"=w405) -> (w442:T5)
        n190 = Bundle By Name(cluster=T3 {"center X"=0.0, "center Y"=0.0, "angle"=0.0, "width"=0.0, "height"=0.0, "# pixels"=0, "# lines"=0} ("Scanfield"), "center X"=w433, "center Y"=w432, "angle"=w431, "width"=w430, "height"=w429, "# lines"=w426, "# pixels"=w427) -> (w428:T3)
        n191 = Bundle("stripped path"=w439, "name"=w438) -> (w437:cluster{"stripped path":path, "name":string})  [unwired: 1 in]
        n192 = call <userlib>:"Save sxm File.vi"("Auto file naming? (T)"=FALSE, "Scanfield"=w428, "Scan param"=w442, "error in (no error)"=w436, "Channels data"=w446, "Channels config"=T4 [{"Name"="Z (m)", "Calibration"=1.0, "Offset"=0.0, "Channel index"=0}], "Filename control"=w437) -> ("error out"=w414:errorcluster)  [unwired: 2 in, 2 out]
        n193 = Strip Path(path=w409) -> (stripped path=w416:path)  [unwired: 1 out]
        n194 = call <userlib>:"Get Session Path.vi"("error in (no error)"=w414, "Application ref in"=w413) -> ("error out"=w410:errorcluster, "Session path"=w412:path, "Application ref out"=w393:refnum<vi>)  [unwired: 7 in]
        n195 = Path To String(path=w409) -> (string=w408:string)
        n196 = Strip Path(path=w416) -> (stripped path=w394:path)  [unwired: 1 out]
        n197 = call "SXM.vi"("Path"=w412, "Delete"=FALSE, "error in"=w410) -> ("error out"=w391:errorcluster)  [unwired: 7 in]
        n198 = call <userlib>:"Set Session Path.vi"("error in (no error)"=w391, "Session Folder"=w394, "Application ref in"=w393) -> ("error out"=w390:errorcluster, "Application ref out"=w392:refnum<vi>)  [unwired: 7 in]
        n199 = Format Date/Time String(time format string (%c)=" Finished at %y%m%d - %H%M%S ", seconds (now)=w405) -> (date/time string=w404:string)  [unwired: 1 in]
        n200 = Concatenate Strings(w408, "\r\n", w404) -> (w407:string)
        n201 = Search and Replace String(input string="Email when finished", search string="@") -> (number of replacements=w400:i32)  [unwired: 6 in, 3 out]
        n202 = Greater Than 0?(x=w400) -> (x > 0?=w399:bool)
        n203 = case shown="True" w399 {
          tunnel: w390 -> [_ w454]
          tunnel: w407 -> [_ w452]
          tunnel: "Email when finished" -> [_ w451]
          frame False {
          }
          frame True {
            n204 = call "Send Email"("error in"=w454, "Message"=w452, "Subject"="Grid Finished", "Recipients"=w451) -> ()  [unwired: 7 in, 1 out]
          }
        }
        n205 = call <userlib>:"BiasSpectroscopy SetProperties.vi"("Application ref in"=w392, "Z-Controller hold (no change)"=enum16{"no change", "on", "off"}."on") -> ("Application ref out"=w397:refnum<vi>)  [unwired: 12 in, 1 out]
        n206 = call <userlib>:"TipLift Set.vi"("TipLift (m)"=sgl 0.0, "Application ref in"=w397) -> ("Application ref out"=w396:refnum<vi>)  [unwired: 8 in, 1 out]
      }
    }
    "Error out" <- w43
    "Points taken" <- w11
    "X Offset" <- w10
    "Y Offset" <- w9
  }
